vi "Run Async CloseApp.vi"(8 "Error In":errorcluster, 11 "Core in":refnum<class "Core.lvclass">) -> (3 "Core out":refnum<class "Core.lvclass">)   [LabVIEW 2019, in "Core.lvlib" / "Core.lvclass"]
uses:
  Core.lvclass
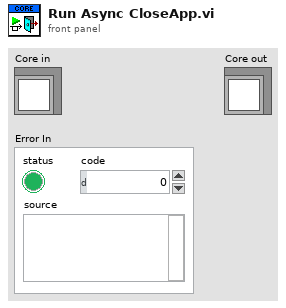
[diagram p1: front panel]
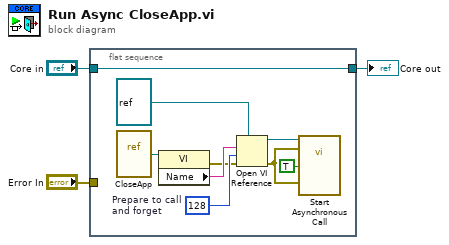
[diagram p0: block diagram]
diagram:
  n1 = flat-sequence {
    tunnel: "Error In" -> [_]
    tunnel: "Core in" -> [w4]
    tunnel: [w4] -> w3
    frame #0 {
      w6 = 128  # Prepare to call and forget
      n2 = vi-ref "CloseApp.vi"() -> (w12:refnum<vi>)
      n3 = property class="VI"(reference=w12) -> (error out=w5:errorcluster, "Name"=w8:string)  [unwired: 1 in, 1 out]
      n4 = Open VI Reference(type specifier VI Refnum (for type only)=refnum<vi> refnum, vi path=w8, options=w6, error in (no error)=w5) -> (vi reference=w11:refnum<vi>, error out=w10:errorcluster)  [unwired: 2 in]
      n5 = call-by-ref "Start Asynchronous Call"(reference=w11, error in=w10, "Error In"=w10, "Show Front Panel?"=TRUE) -> ()  [unwired: 2 in, 2 out]
    }
  }
  "Core out" <- w3
